vi "MarginRight.vi"(1 "输入":dbl[][](array[numeric])) -> (0 "输出":dbl)   [LabVIEW 2016]
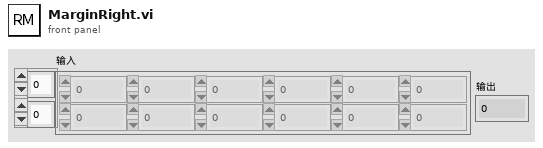
[diagram p1: front panel]
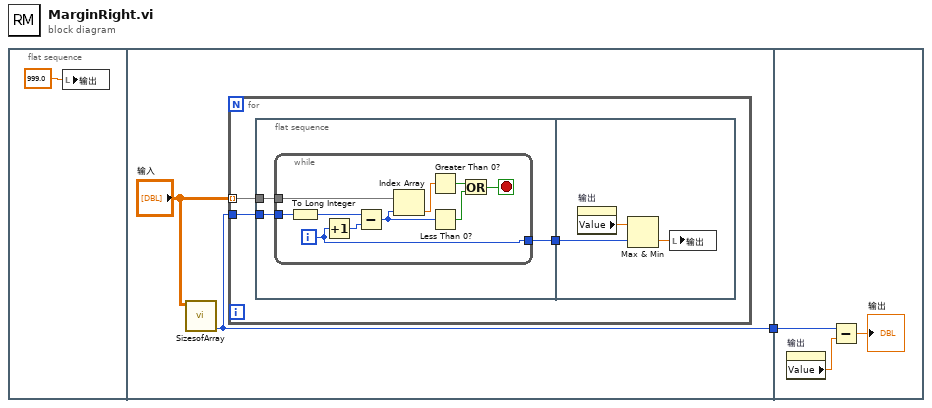
[diagram p0: block diagram]
diagram:
  n1 = flat-sequence {
    tunnel: [w3] -> w1
    tunnel: w1 -> [w24]
    frame #0 {
      n2 = local write "输出"(999.0) -> ()
    }
    frame #1 {
      n3 = call "SizesofArray.vi"("数组"="输入") -> ("NumCols_r"=w3:i32)  [unwired: 7 in, 3 out]
      n4 = for {
        tunnel: "输入" -> [w7] mode=indexing
        tunnel: w3 -> [w5]
        n5 = flat-sequence {
          tunnel: w7 -> [w9]
          tunnel: [w10] -> w6
          tunnel: w5 -> [w8]
          tunnel: w6 -> [w21]
          frame #0 {
            n6 = while {
              tunnel: w9 -> [w20]
              tunnel: [w19] -> w10
              tunnel: w8 -> [w11]
              i -> [w19]
              stop <- w15 stop-if-true
              n7 = To Long Integer(number=w11) -> (32bit integer=w12:i32)
              n8 = Increment(x=w19) -> (x+1=w18:i32)
              n9 = Subtract(x=w12, y=w18) -> (x-y=w16:i32)
              n10 = Index Array(array=w20, index=w16) -> (element=w17:dbl)
              n11 = Greater Than 0?(x=w17) -> (x > 0?=w14:bool)
              n12 = Less Than 0?(x=w16) -> (x < 0?=w13:bool)
              n13 = Or(x=w14, y=w13) -> (x .or. y?=w15:bool)
            }
          }
          frame #1 {
            n14 = property on="输出" class="DigNum (严格)"() -> ("Value"=w22:dbl)  [unwired: 2 in, 2 out]
            n15 = Max & Min(x=w22, y=w21) -> (min(x,y)=w23:dbl)  [unwired: 1 out]
            n16 = local write "输出"(w23) -> ()
          }
        }
      }
    }
    frame #2 {
      n17 = property on="输出" class="DigNum (严格)"() -> ("Value"=w25:dbl)  [unwired: 2 in, 2 out]
      n18 = Subtract(x=w24, y=w25) -> (x-y=→"输出":dbl)
    }
  }
